vi "Autonomous.vi"() -> ()   [LabVIEW 2023]
doc: "This VI starts when autonomous period begins, and will automatically be terminated when it ends. You can carry out timed or sensor driven operations directly to I/O or to subsystems without needing to return to the caller."
uses:
  MHZLib/Variables and Definitions/Auto_Values.ctl
  f91a2575-bbb2-4fc1-b202-6733d6dd800e.vi
  <vilib>/Rock Robotics/WPI/Utilities/WPI_GetSetVariantRefNum.vi
  <vilib>/Rock Robotics/Network Tables/NT Read String.vi
  <vilib>/Rock Robotics/Network Tables/NT Read Variant.vi
  MHZLib/Variables and Definitions/Robot Global Data.vi
  <vilib>/addons/control/pid/pid.llb/PID (DBL).vi
  <vilib>/addons/control/pid/NI_PID_pid.lvlib
panel:
  in  "PID rot":T1={"proportional gain (Kc)"=1.0, "integral time (Ti, min)"=0.01, "derivative time (Td, min)"=0.0} {"derivative time (Td, min)" format="%.3f"; "integral time (Ti, min)" format="%.3f"; "proportional gain (Kc)" format="%.3f"}
  in  "PID y":T1={"proportional gain (Kc)"=1.0, "integral time (Ti, min)"=0.01, "derivative time (Td, min)"=0.0} {"derivative time (Td, min)" format="%.3f"; "integral time (Ti, min)" format="%.3f"; "proportional gain (Kc)" format="%.3f"}
  in  "PID x":T1={"proportional gain (Kc)"=1.0, "integral time (Ti, min)"=0.01, "derivative time (Td, min)"=0.0} {"derivative time (Td, min)" format="%.3f"; "integral time (Ti, min)" format="%.3f"; "proportional gain (Kc)" format="%.3f"}
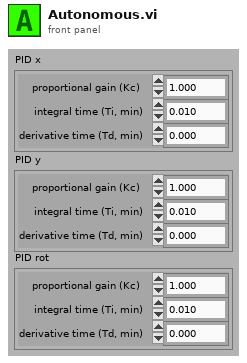
[diagram p1: front panel]
types:
  T1 = cluster{"proportional gain (Kc)":dbl, "integral time (Ti, min)":dbl, "derivative time (Td, min)":dbl}
  T2 = typedef "Auto_Values.ctl" = cluster{"X Pos":dbl, "Y Pos":dbl, "Heading (Deg)":dbl, "Strafe Throttle":dbl, "Rot Throtle (Rad/s)":dbl, "Strafe Tol (Ft)":dbl, "Rotation Tol (Deg)":dbl, "Shooter Pos":enum16{"Hold", "Travel", "Speaker", "Amp"}, "Intake":enum16{"Off", "Front", "Center", "Out"}, "Auto Aim":enum16{"Off", "Aim", "Aim & Shoot"}, "Shooter Throttle":dbl, "Wait (s)":dbl, "Lift":enum16{"Off", "Up", "Down"}, "Shoot?":bool}
  T3 = typedef "WPI_JoystickDevRef.ctl" = cluster{"Device":T4}
  T4 = typedef "WPI_JoystickDeviceEnum.ctl" = enum16{"USB 0", "USB 1", "USB 2", "USB 3", "USB 4", "USB 5"}
  T5 = typedef "WPI_DriverStationAllianceInfo.ctl" = enum16{"Red", "Blue", "Invalid"}
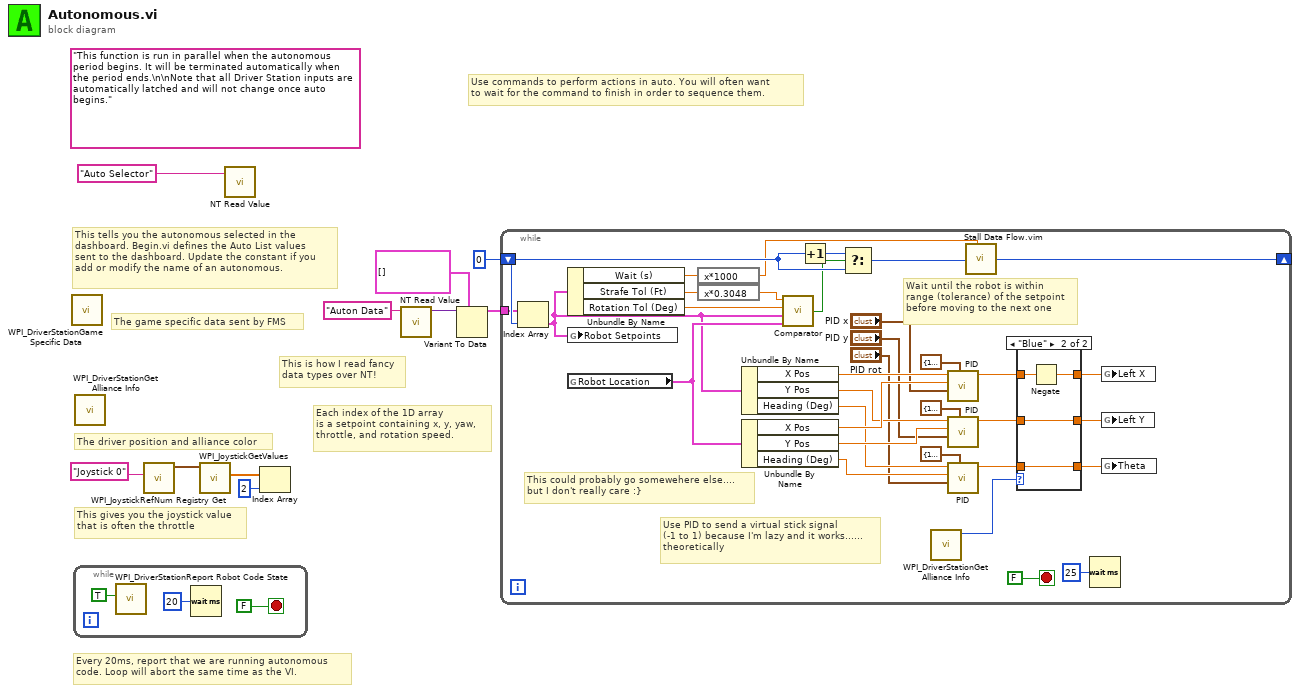
[diagram p0: block diagram]
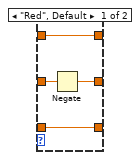
[diagram p2: hidden frame]
diagram:
  (unwired) "This function is run in parallel when the autonomous period begins. It will be terminated automatically when the period ends.\n\nNote that all Driver Station inputs are automatically latched and will not change once auto begins."
  # "This is how I read fancy\ndata types over NT!"
  # "Each index of the 1D array\nis a setpoint containing x, y, yaw,\nthrottle, and rotation speed."
  # "The game specific data sent by FMS"
  # "This tells you the autonomous selected in the \ndashboard. Begin.vi defines the Auto List values\nsent to the dashboard. Update the constant if you\nadd or modify the name of an autonomous."
  # "Every 20ms, report that we are running autonomous\ncode. Loop will abort the same time as the VI."
  # "This gives you the joystick value\nthat is often the throttle"
  # "Use commands to perform actions in auto. You will often want\nto wait for the command to finish in order to sequence them."
  # "The driver position and alliance color"
  n1 = call <vilib>:"WPI_DriverStationGame Specific Data.vi"() -> ()  [unwired: 11 in, 1 out]
  n2 = while {
    stop <- FALSE stop-if-true
    n3 = call <vilib>:"WPI_DriverStationReport Robot Code State.vi"("Autonomous"=TRUE) -> ()  [unwired: 10 in, 1 out]
    n4 = Wait (ms)(milliseconds to wait=u32 20) -> ()  [unwired: 1 out]
  }
  n5 = call <vilib>:"WPI_DriverStationGet Alliance Info.vi"() -> ()  [unwired: 12 out]
  n6 = call <vilib>:"WPI_JoystickRefNum Registry Get.vi"("refnum name"="Joystick 0") -> ("JoystickDevRef"=w9:T3)  [unwired: 1 in, 9 out]
  n7 = call <vilib>:"WPI_JoystickGetValues.vi"("JoystickDevRef"=w9) -> ("Axes"=w8:dbl[])  [unwired: 6 in, 4 out]
  n8 = call-poly <vilib>:"NT Read Value.vi"("name"="Auto Selector" ("Name")) -> ()  [unwired: 8 in, 3 out]
  n9 = Index Array(array=w8, index=2) -> ()  [unwired: 1 out]
  n10 = call-poly <vilib>:"NT Read Value.vi"("name"="Auton Data") -> ("Variant"=w4:variant)  [unwired: 9 in, 1 out]
  n11 = Variant To Data(type=T2[] [] ("appended array"), Variant=w4) -> (data=w1:T2[])  [unwired: 1 in, 1 out]
  n12 = while {
    shift-right: [w25] -> _
    shift-left: 0 ("index") -> [w43]
    tunnel: w1 -> [w39]
    stop <- FALSE stop-if-true
    # "This could probably go somewehere else....\nbut I don't really care :}"
    # "Use PID to send a virtual stick signal\n(-1 to 1) because I'm lazy and it works......\ntheoretically"
    # "Wait until the robot is within\nrange (tolerance) of the setpoint\nbefore moving to the next one"
    n13 = Index Array(array=w39, index=w43) -> (element=w26:T2)
    n14 = Unbundle By Name(w26) -> ("Wait (s)"=w23:dbl, "Strafe Tol (Ft)"=w27:dbl, "Rotation Tol (Deg)"=w28:dbl)
    n15 = global write "Robot Global Data.vi" "Robot Setpoints"(w26) -> ()
    n16 = global read "Robot Global Data.vi" "Robot Location"() -> (w38:T2)
    n17 = expression code="x*1000"(w23) -> (w22:dbl)
    n18 = expression code="x*0.3048"(w27) -> (w21:dbl)
    n19 = Unbundle By Name(w26) -> ("X Pos"=w37:dbl, "Y Pos"=w33:dbl, "Heading (Deg)"=w32:dbl)
    n20 = Unbundle By Name(w38) -> ("X Pos"=w36:dbl, "Y Pos"=w35:dbl, "Heading (Deg)"=w34:dbl)
    n21 = call "Comparator.vi"("Current Location"=w38, "Target Location"=w26, "Rotate Tolerance"=w28, "Strafe Tolerance"=w21) -> ("In range?"=w42:bool)
    n22 = Increment(x=w43) -> (x+1=w44:i32)
    n23 = Select(t=w44, s=w42, f=w43) -> (s? t:f=w24:i32)
    n24 = call <vilib>:"WPI_DriverStationGet Alliance Info.vi"() -> ("Alliance"=w19:T5)  [unwired: 6 in, 5 out]
    n25 = call-poly <vilib>:"PID.vi"("output range"=cluster{"output high":dbl, "output low":dbl} {"output high"=1.0, "output low"=-1.0}, "PID gains"="PID x", "process variable"=w36, "setpoint"=w37) -> ("output"=w17:dbl)  [unwired: 6 in, 1 out]
    n26 = call-poly <vilib>:"PID.vi"("output range"=cluster{"output high":dbl, "output low":dbl} {"output high"=1.0, "output low"=-1.0}, "PID gains"="PID y", "process variable"=w35, "setpoint"=w33) -> ("output"=w18:dbl)  [unwired: 6 in, 1 out]
    n27 = call-poly <vilib>:"PID.vi"("output range"=cluster{"output high":dbl, "output low":dbl} {"output high"=1.0, "output low"=-1.0}, "PID gains"="PID rot", "process variable"=w34, "setpoint"=w32) -> ("output"=w20:dbl)  [unwired: 6 in, 1 out]
    n28 = call "Stall Data Flow.vim"("value in"=w24, "milliseconds to wait"=w22) -> ("value out"=w25:i32)  [unwired: 1 out]
    n29 = case shown="\"Blue\"" w19 {
      tunnel: [w51 w55] -> w14
      tunnel: w20 -> [w51 w55]
      tunnel: w18 -> [w50 w54]
      tunnel: w17 -> [w49 w53]
      tunnel: [w50 w52] -> w16
      tunnel: [w48 w53] -> w15
      frame "Red", Default {
        n30 = Negate(x=w49) -> (-x=w48:dbl)
      }
      frame "Blue" {
        n31 = Negate(x=w54) -> (-x=w52:dbl)
      }
    }
    n32 = Wait (ms)(milliseconds to wait=u32 25) -> ()  [unwired: 1 out]
    n33 = global write "Robot Global Data.vi" "Left X"(w16) -> ()
    n34 = global write "Robot Global Data.vi" "Left Y"(w15) -> ()
    n35 = global write "Robot Global Data.vi" "Theta"(w14) -> ()
  }
